vi "PXF4_set_hysteresis.vi"(8 "error in":errorcluster, 10 "hysteresis":i16=1, 11 "Modbus Master in":refnum<class "Modbus Master.lvclass">) -> (0 "error out":errorcluster, 3 "Modbus Master out":refnum<class "Modbus Master.lvclass">)   [LabVIEW 2019]
uses:
  <vilib>/NI/Modbus Library/API/Master/Modbus Master.lvclass
panel:
  out "value":dbl
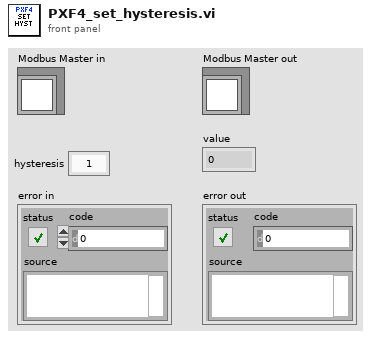
[diagram p1: front panel]
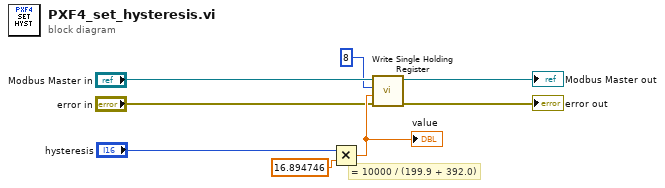
[diagram p0: block diagram]
diagram:
  # "= 10000 / (199.9 + 392.0)"
  n1 = Multiply(x="hysteresis", y=16.894746) -> (x*y=w7:dbl)
  "value" <- w7
  n2 = call-dynamic "Write Single Holding Register.vi"("error in"="error in", "register to write"=w7, "address"=u16 8, "Modbus master in"="Modbus Master in") -> ("error out"=→"error out":errorcluster, "Modbus master out"=→"Modbus Master out":refnum<class "Modbus Master.lvclass">)  [unwired: 6 in]
